vi "GetConfig.vi"(10 "Cameras":T1[](array[typedef])) -> ()   [LabVIEW 2014]
uses:
  Controls/CamView_Properties.ctl
panel:
  in  "Error IN":errorcluster
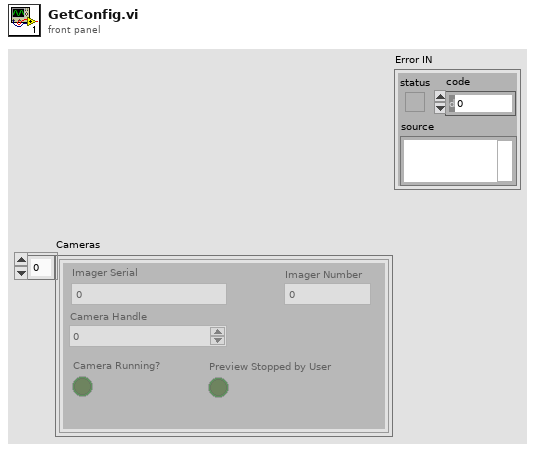
[diagram p1: front panel]
types:
  T1 = typedef "CamView_Properties.ctl" = cluster{"Imager Serial":u32, "Camera Handle":u32, "Camera Running?":bool, "Preview Stopped by User":bool, "Imager Number":u32}
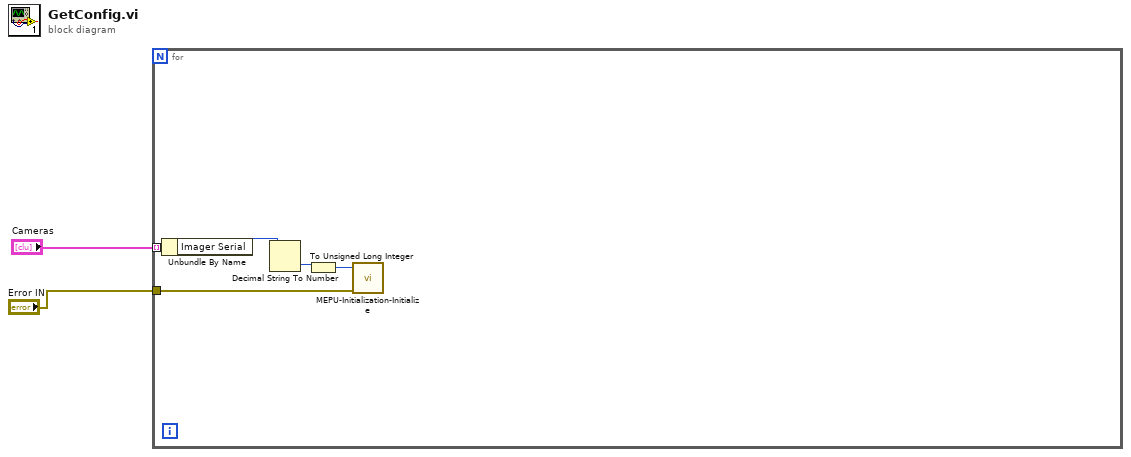
[diagram p0: block diagram]
diagram:
  n1 = for {
    tunnel: "Cameras" -> [w7] mode=indexing
    tunnel: "Error IN" -> [w3]
    n2 = Unbundle By Name(w7) -> ("Imager Serial"=w6:u32)
    n3 = Decimal String To Number(string=w6) -> (number=w5:i32)  [unwired: 2 in, 1 out]
    n4 = To Unsigned Long Integer(number=w5) -> (unsigned 32bit integer=w4:u32)
    n5 = call <vilib>:"MEPU-Initialization-Initialize.vi"("uSerialNumber IN"=w4, "Error IN"=w3) -> ()  [unwired: 14 out]
  }
